vi "var_num_v4.vi"() -> ()   [LabVIEW 2009]
panel:
  out "Gauge":dbl(knob)=200.54901947339192 scale=0.0..1000.0
  out "Slide":dbl(slide)=200.54901947339192 scale=0.0..1000.0
  out "Numeric":dbl=200.54901947339192
  in  "Ui":dbl(slide)=200.54901947339192 scale=0.0..1000.0
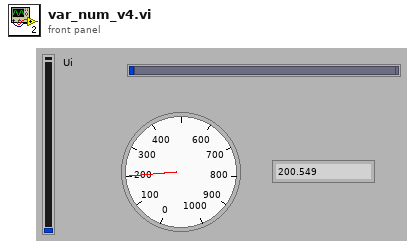
[diagram p1: front panel]
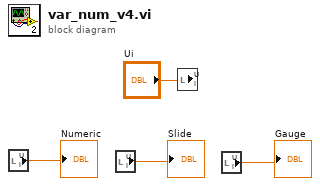
[diagram p0: block diagram]
diagram:
  n1 = local read "Ui"() -> (→"Numeric":dbl)
  n2 = local read "Ui"() -> (→"Slide":dbl)
  n3 = local write "Ui"("Ui") -> ()
  n4 = local read "Ui"() -> (→"Gauge":dbl)
